vi "FaulhaberV3-Ascii_V1.vi"() -> (1 "searchnames":string[](array[string]), 2 "ID":u32[](array[numeric]), 3 "Faulhaber Objects":T3(array[cluster]))   [LabVIEW 2011] (continued)
of entries", "type"=enum."U8", "rw"=enum."ro", "lowLimit"="", "highLimit"="", "Default"="5", "Kommentart"=""}, {"ID"=594608129, "Name"="Trace buffer_Trace state", "type"=enum."U16", "rw"=enum."ro", "lowLimit"="", "highLimit"="", "Default"="", "Kommentart"=""}, {"ID"=594673664, "Name"="Logic trigger configuration_Number of entries", "type"=enum."U8", "rw"=enum."ro", "lowLimit"="", "highLimit"="", "Default"="2", "Kommentart"=""}, {"ID"=594673665, "Name"="Logic trigger configuration_Logic trigger AND mask", "type"=enum."U32", "rw"=enum."rw", "lowLimit"="0", "highLimit"="4294967295", "Default"="0x00", "Kommentart"=""}, {"ID"=594673666, "Name"="Logic trigger configuration_Logic trigger OR mask", "type"=enum."U32", "rw"=enum."rw", "lowLimit"="0", "highLimit"="4294967295", "Default"="0x00", "Kommentart"=""}, {"ID"=594739200, "Name"="Event trigger configuration_Number of entries", "type"=enum."U8", "rw"=enum."ro", "lowLimit"="", "highLimit"="", "Default"="1", "Kommentart"=""}, {"ID"=594739201, "Name"="Event trigger configuration_Event trigger event selection", "type"=enum."U16", "rw"=enum."unknown", "lowLimit"="", "highLimit"="", "Default"="", "Kommentart"=""}, {"ID"=594804736, "Name"="Event flag configuration_Number of entries", "type"=enum."U8", "rw"=enum."ro", "lowLimit"="", "highLimit"="", "Default"="2", "Kommentart"=""}, {"ID"=594804737, "Name"="Event flag configuration_Event flag set mask", "type"=enum."U16", "rw"=enum."rw", "lowLimit"="0", "highLimit"="65535", "Default"="0x0", "Kommentart"=""}, {"ID"=594804738, "Name"="Event flag configuration_Event flag reset mask", "type"=enum."U16", "rw"=enum."rw", "lowLimit"="0", "highLimit"="65535", "Default"="0x0", "Kommentart"=""}, {"ID"=595066880, "Name"="Trace channel configuration_Number of entries", "type"=enum."U8", "rw"=enum."ro", "lowLimit"="", "highLimit"="", "Default"="23", "Kommentart"=""}, {"ID"=595066881, "Name"="Trace channel configuration_Channel 1 filter time", "type"=enum."U16", "rw"=enum."rw", "lowLimit"="0", "highLimit"="65535", "Default"="0", "Kommentart"=""}, {"ID"=595066882, "Name"="Trace channel configuration_Channel 1 sample time", "type"=enum."U16", "rw"=enum."rw", "lowLimit"="0", "highLimit"="65535", "Default"="1", "Kommentart"=""}, {"ID"=595066883, "Name"="Trace channel configuration_Channel 1 number of samples", "type"=enum."U16", "rw"=enum."rw", "lowLimit"="0", "highLimit"="65535", "Default"="512", "Kommentart"=""}, {"ID"=595066884, "Name"="Trace channel configuration_Channel 1 monitoring values", "type"=enum."U16", "rw"=enum."rw", "lowLimit"="0", "highLimit"="0x003F", "Default"="0", "Kommentart"=""}, {"ID"=595066885, "Name"="Trace channel configuration_Channel 1 start event selection", "type"=enum."U8", "rw"=enum."unknown", "lowLimit"="", "highLimit"="", "Default"="", "Kommentart"=""}, {"ID"=595066886, "Name"="Trace channel configuration_Channel 1 update event selection", "type"=enum."U8", "rw"=enum."unknown", "lowLimit"="", "highLimit"="", "Default"="", "Kommentart"=""}, {"ID"=595066887, "Name"="Trace channel configuration_Channel 1 number of eval-cycles", "type"=enum."U32", "rw"=enum."rw", "lowLimit"="0", "highLimit"="4294967295", "Default"="0", "Kommentart"=""}, {"ID"=595066894, "Name"="Trace channel configuration_Channel 1 number of turnovers", "type"=enum."U32", "rw"=enum."ro", "lowLimit"="", "highLimit"="", "Default"="", "Kommentart"=""}, {"ID"=595066895, "Name"="Trace channel configuration_Channel 1 done", "type"=enum."U8", "rw"=enum."ro", "lowLimit"="", "highLimit"="", "Default"="", "Kommentart"=""}, {"ID"=595066896, "Name"="Trace channel configuration_Channel 1 abs min value", "type"=enum."S32", "rw"=enum."ro", "lowLimit"="", "highLimit"="", "Default"="2147483647", "Kommentart"=""}, {"ID"=595066897, "Name"="Trace channel configuration_Channel 1 abs max value", "type"=enum."S32", "rw"=enum."ro", "lowLimit"="", "highLimit"="", "Default"="-2147483648", "Kommentart"=""}, {"ID"=595066898, "Name"="Trace channel configuration_Channel 1 minimum", "type"=enum."S32", "rw"=enum."ro", "lowLimit"="", "highLimit"="", "Default"="", "Kommentart"=""}, {"ID"=595066899, "Name"="Trace channel configuration_Channel 1 maximum", "type"=enum."S32", "rw"=enum."ro", "lowLimit"="", "highLimit"="", "Default"="", "Kommentart"=""}, {"ID"=595066900, "Name"="Trace channel configuration_Channel 1 mean value", "type"=enum."S32", "rw"=enum."ro", "lowLimit"="", "highLimit"="", "Default"="", "Kommentart"=""}, {"ID"=595066901, "Name"="Trace channel configuration_Channel 1 rms value", "type"=enum."S32", "rw"=enum."ro", "lowLimit"="", "highLimit"="", "Default"="", "Kommentart"=""}, {"ID"=595066902, "Name"="Trace channel configuration_Channel 1 period time", "type"=enum."U32", "rw"=enum."ro", "lowLimit"="", "highLimit"="", "Default"="", "Kommentart"=""}, {"ID"=595066903, "Name"="Trace channel configuration_Channel 1 sigma", "type"=enum."S32", "rw"=enum."ro", "lowLimit"="", "highLimit"="", "Default"="", "Kommentart"=""}, {"ID"=595132416, "Name"="Trace channel configuration_Number of entries", "type"=enum."U8", "rw"=enum."ro", "lowLimit"="", "highLimit"="", "Default"="23", "Kommentart"=""}, {"ID"=595132417, "Name"="Trace channel configuration_Channel 2 filter time", "type"=enum."U16", "rw"=enum."rw", "lowLimit"="0", "highLimit"="65535", "Default"="0", "Kommentart"=""}, {"ID"=595132418, "Name"="Trace channel configuration_Channel 2 sample time", "type"=enum."U16", "rw"=enum."rw", "lowLimit"="0", "highLimit"="65535", "Default"="1", "Kommentart"=""}, {"ID"=595132419, "Name"="Trace channel configuration_Channel 2 number of samples", "type"=enum."U16", "rw"=enum."rw", "lowLimit"="0", "highLimit"="65535", "Default"="512", "Kommentart"=""}, {"ID"=595132420, "Name"="Trace channel configuration_Channel 2 monitoring values", "type"=enum."U16", "rw"=enum."rw", "lowLimit"="0", "highLimit"="0x003F", "Default"="0", "Kommentart"=""}, {"ID"=595132421, "Name"="Trace channel configuration_Channel 2 startevent selection", "type"=enum."U8", "rw"=enum."unknown", "lowLimit"="", "highLimit"="", "Default"="", "Kommentart"=""}, {"ID"=595132422, "Name"="Trace channel configuration_Channel 2 update event selection", "type"=enum."U8", "rw"=enum."unknown", "lowLimit"="", "highLimit"="", "Default"="", "Kommentart"=""}, {"ID"=595132423, "Name"="Trace channel configuration_Channel 2 number of eval-cycles", "type"=enum."U32", "rw"=enum."rw", "lowLimit"="0", "highLimit"="4294967295", "Default"="0", "Kommentart"=""}, {"ID"=595132430, "Name"="Trace channel configuration_Channel 2 number of turn-overs", "type"=enum."U32", "rw"=enum."ro", "lowLimit"="", "highLimit"="", "Default"="", "Kommentart"=""}, {"ID"=595132431, "Name"="Trace channel configuration_Channel 2 done", "type"=enum."U8", "rw"=enum."ro", "lowLimit"="", "highLimit"="", "Default"="", "Kommentart"=""}, {"ID"=595132432, "Name"="Trace channel configuration_Channel 2 abs min value", "type"=enum."S32", "rw"=enum."ro", "lowLimit"="", "highLimit"="", "Default"="2147483647", "Kommentart"=""}, {"ID"=595132433, "Name"="Trace channel configuration_Channel 2 abs max value", "type"=enum."S32", "rw"=enum."ro", "lowLimit"="", "highLimit"="", "Default"="-2147483648", "Kommentart"=""}, {"ID"=595132434, "Name"="Trace channel configuration_Channel 2 minimum", "type"=enum."S32", "rw"=enum."ro", "lowLimit"="", "highLimit"="", "Default"="", "Kommentart"=""}, {"ID"=595132435, "Name"="Trace channel configuration_Channel 2 maximum", "type"=enum."S32", "rw"=enum."ro", "lowLimit"="", "highLimit"="", "Default"="", "Kommentart"=""}, {"ID"=595132436, "Name"="Trace channel configuration_Channel 2 mean value", "type"=enum."S32", "rw"=enum."ro", "lowLimit"="", "highLimit"="", "Default"="", "Kommentart"=""}, {"ID"=595132437, "Name"="Trace channel configuration_Channel 2 rms value", "type"=enum."S32", "rw"=enum."ro", "lowLimit"="", "highLimit"="", "Default"="", "Kommentart"=""}, {"ID"=595132438, "Name"="Trace channel configuration_Channel 2 period time", "type"=enum."U32", "rw"=enum."ro", "lowLimit"="", "highLimit"="", "Default"="", "Kommentart"=""}, {"ID"=595132439, "Name"="Trace channel configuration_Channel 2 sigma", "type"=enum."S32", "rw"=enum."ro", "lowLimit"="", "highLimit"="", "Default"="", "Kommentart"=""}, {"ID"=595197952, "Name"="Trace channel configuration_Number of entries", "type"=enum."U8", "rw"=enum."ro", "lowLimit"="", "highLimit"="", "Default"="23", "Kommentart"=""}, {"ID"=595197953, "Name"="Trace channel configuration_Channel 3 filter time", "type"=enum."U16", "rw"=enum."rw", "lowLimit"="0", "highLimit"="65535", "Default"="0", "Kommentart"=""}, {"ID"=595197954, "Name"="Trace channel configuration_Channel 3 sample time", "type"=enum."U16", "rw"=enum."rw", "lowLimit"="0", "highLimit"="65535", "Default"="1", "Kommentart"=""}, {"ID"=595197955, "Name"="Trace channel configuration_Channel 3 number of samples", "type"=enum."U16", "rw"=enum."rw", "lowLimit"="0", "highLimit"="65535", "Default"="512", "Kommentart"=""}, {"ID"=595197956, "Name"="Trace channel configuration_Channel 3 monitoring values", "type"=enum."U16", "rw"=enum."rw", "lowLimit"="0", "highLimit"="0x003F", "Default"="0", "Kommentart"=""}, {"ID"=595197957, "Name"="Trace channel configuration_Channel 3 start event selection", "type"=enum."U8", "rw"=enum."unknown", "lowLimit"="", "highLimit"="", "Default"="", "Kommentart"=""}, {"ID"=595197958, "Name"="Trace channel configuration_Channel 3 update event selection", "type"=enum."U8", "rw"=enum."unknown", "lowLimit"="", "highLimit"="", "Default"="", "Kommentart"=""}, {"ID"=595197959, "Name"="Trace channel configuration_Channel 3 number of eval-cycles", "type"=enum."U32", "rw"=enum."rw", "lowLimit"="0", "highLimit"="4294967295", "Default"="0", "Kommentart"=""}, {"ID"=595197966, "Name"="Trace channel configuration_Channel 3 number of turn-overs", "type"=enum."U32", "rw"=enum."ro", "lowLimit"="", "highLimit"="", "Default"="", "Kommentart"=""}, {"ID"=595197967, "Name"="Trace channel configuration_Channel 3 done", "type"=enum."U8", "rw"=enum."ro", "lowLimit"="", "highLimit"="", "Default"="", "Kommentart"=""}, {"ID"=595197968, "Name"="Trace channel configuration_Channel 3 abs min value", "type"=enum."S32", "rw"=enum."ro", "lowLimit"="", "highLimit"="", "Default"="2147483647", "Kommentart"=""}, {"ID"=595197969, "Name"="Trace channel configuration_Channel 3 abs max value", "type"=enum."S32", "rw"=enum."ro", "lowLimit"="", "highLimit"="", "Default"="-2147483648", "Kommentart"=""}, {"ID"=595197970, "Name"="Trace channel configuration_Channel 3 minimum", "type"=enum."S32", "rw"=enum."ro", "lowLimit"="", "highLimit"="", "Default"="", "Kommentart"=""}, {"ID"=595197971, "Name"="Trace channel configuration_Channel 3 maximum", "type"=enum."S32", "rw"=enum."ro", "lowLimit"="", "highLimit"="", "Default"="", "Kommentart"=""}, {"ID"=595197972, "Name"="Trace channel configuration_Channel 3 mean value", "type"=enum."S32", "rw"=enum."ro", "lowLimit"="", "highLimit"="", "Default"="", "Kommentart"=""}, {"ID"=595197973, "Name"="Trace channel configuration_Channel 3 rms value", "type"=enum."S32", "rw"=enum."ro", "lowLimit"="", "highLimit"="", "Default"="", "Kommentart"=""}, {"ID"=595197974, "Name"="Trace channel configuration_Channel 3 period time", "type"=enum."U32", "rw"=enum."ro", "lowLimit"="", "highLimit"="", "Default"="", "Kommentart"=""}, {"ID"=595197975, "Name"="Trace channel configuration_Channel 3 sigma", "type"=enum."S32", "rw"=enum."ro", "lowLimit"="", "highLimit"="", "Default"="", "Kommentart"=""}, {"ID"=595263488, "Name"="Trace channel configuration_Number of entries", "type"=enum."U8", "rw"=enum."ro", "lowLimit"="", "highLimit"="", "Default"="23", "Kommentart"=""}, {"ID"=595263489, "Name"="Trace channel configuration_Channel 4 filter time", "type"=enum."U16", "rw"=enum."rw", "lowLimit"="0", "highLimit"="65535", "Default"="0", "Kommentart"=""}, {"ID"=595263490, "Name"="Trace channel configuration_Channel 4 sample time", "type"=enum."U16", "rw"=enum."rw", "lowLimit"="0", "highLimit"="65535", "Default"="1", "Kommentart"=""}, {"ID"=595263491, "Name"="Trace channel configuration_Channel 4 number of samples", "type"=enum."U16", "rw"=enum."rw", "lowLimit"="0", "highLimit"="65535", "Default"="512", "Kommentart"=""}, {"ID"=595263492, "Name"="Trace channel configuration_Channel 4 monitoring values", "type"=enum."U16", "rw"=enum."rw", "lowLimit"="0", "highLimit"="0x003F", "Default"="0", "Kommentart"=""}, {"ID"=595263493, "Name"="Trace channel configuration_Channel 4 start event selection", "type"=enum."U8", "rw"=enum."unknown", "lowLimit"="", "highLimit"="", "Default"="", "Kommentart"=""}, {"ID"=595263494, "Name"="Trace channel configuration_Channel 4 update event selection", "type"=enum."U8", "rw"=enum."unknown", "lowLimit"="", "highLimit"="", "Default"="", "Kommentart"=""}, {"ID"=595263495, "Name"="Trace channel configuration_Channel 4 number of eval-cycles", "type"=enum."U32", "rw"=enum."rw", "lowLimit"="0", "highLimit"="4294967295", "Default"="0", "Kommentart"=""}, {"ID"=595263502, "Name"="Trace channel configuration_Channel 4 number of turn-overs", "type"=enum."U32", "rw"=enum."ro", "lowLimit"="", "highLimit"="", "Default"="", "Kommentart"=""}, {"ID"=595263503, "Name"="Trace channel configuration_Channel 4 done", "type"=enum."U8", "rw"=enum."ro", "lowLimit"="", "highLimit"="", "Default"="", "Kommentart"=""}, {"ID"=595263504, "Name"="Trace channel configuration_Channel 4 abs min value", "type"=enum."S32", "rw"=enum."ro", "lowLimit"="", "highLimit"="", "Default"="2147483647", "Kommentart"=""}, {"ID"=595263505, "Name"="Trace channel configuration_Channel 4 abs max value", "type"=enum."S32", "rw"=enum."ro", "lowLimit"="", "highLimit"="", "Default"="-2147483648", "Kommentart"=""}, {"ID"=595263506, "Name"="Trace channel configuration_Channel 4 minimum", "type"=enum."S32", "rw"=enum."ro", "lowLimit"="", "highLimit"="", "Default"="", "Kommentart"=""}, {"ID"=595263507, "Name"="Trace channel configuration_Channel 4 maximum", "type"=enum."S32", "rw"=enum."ro", "lowLimit"="", "highLimit"="", "Default"="", "Kommentart"=""}, {"ID"=595263508, "Name"="Trace channel configuration_Channel 4 mean value", "type"=enum."S32", "rw"=enum."ro", "lowLimit"="", "highLimit"="", "Default"="", "Kommentart"=""}, {"ID"=595263509, "Name"="Trace channel configuration_Channel 4 rms value", "type"=enum."S32", "rw"=enum."ro", "lowLimit"="", "highLimit"="", "Default"="", "Kommentart"=""}, {"ID"=595263510, "Name"="Trace channel configuration_Channel 4 period time", "type"=enum."U32", "rw"=enum."ro", "lowLimit"="", "highLimit"="", "Default"="", "Kommentart"=""}, {"ID"=595263511, "Name"="Trace channel configuration_Channel 4 sigma", "type"=enum."S32", "rw"=enum."ro", "lowLimit"="", "highLimit"="", "Default"="", "Kommentart"=""}, {"ID"=595591168, "Name"="PRBS generator_Number of entries", "type"=enum."U8", "rw"=enum."ro", "lowLimit"="", "highLimit"="", "Default"="5", "Kommentart"=""}, {"ID"=595591169, "Name"="PRBS generator_Shift register init", "type"=enum."U16", "rw"=enum."rw", "lowLimit"="0", "highLimit"="65535", "Default"="", "Kommentart"=""}, {"ID"=595591170, "Name"="PRBS generator_Gain", "type"=enum."S16", "rw"=enum."rw", "lowLimit"="-32768", "highLimit"="32767", "Default"="", "Kommentart"=""}, {"ID"=595591171, "Name"="PRBS generator_Offset", "type"=enum."S16", "rw"=enum."rw", "lowLimit"="-32768", "highLimit"="32767", "Default"="", "Kommentart"=""}, {"ID"=595591172, "Name"="PRBS generator_Sample rate factor", "type"=enum."U8", "rw"=enum."rw", "lowLimit"="0", "highLimit"="255", "Default"="", "Kommentart"=""}, {"ID"=595591173, "Name"="PRBS generator_Enable", "type"=enum."U8", "rw"=enum."rw", "lowLimit"="0", "highLimit"="255", "Default"="", "Kommentart"=""}, {"ID"=595656704, "Name"="Start up generator_Number of entries", "type"=enum."U8", "rw"=enum."ro", "lowLimit"="", "highLimit"="", "Default"="8", "Kommentart"=""}, {"ID"=595656705, "Name"="Start up generator_Speed threshold", "type"=enum."U16", "rw"=enum."rw", "lowLimit"="0", "highLimit"="65535", "Default"="", "Kommentart"=""}, {"ID"=595656706, "Name"="Start up generator_Timeout time", "type"=enum."U32", "rw"=enum."rw", "lowLimit"="0", "highLimit"="4294967295", "Default"="", "Kommentart"=""}, {"ID"=595656707, "Name"="Start up generator_Target value", "type"=enum."U16", "rw"=enum."rw", "lowLimit"="0", "highLimit"="65535", "Default"="", "Kommentart"=""}, {"ID"=595656708, "Name"="Start up generator_Reset", "type"=enum."U8", "rw"=enum."rw", "lowLimit"="0", "highLimit"="255", "Default"="", "Kommentart"=""}, {"ID"=595656709, "Name"="Start up generator_Enable", "type"=enum."U8", "rw"=enum."rw", "lowLimit"="0", "highLimit"="255", "Default"="", "Kommentart"=""}, {"ID"=595656710, "Name"="Start up generator_Ready", "type"=enum."U32", "rw"=enum."rw", "lowLimit"="0", "highLimit"="4294967295", "Default"="", "Kommentart"=""}, {"ID"=595656711, "Name"="Start up generator_TimeThreshold", "type"=enum."U32", "rw"=enum."rw", "lowLimit"="0", "highLimit"="4294967295", "Default"="", "Kommentart"=""}, {"ID"=595656712, "Name"="Start up generator_Iteration", "type"=enum."U32", "rw"=enum."rw", "lowLimit"="0", "highLimit"="4294967295", "Default"="", "Kommentart"=""}, {"ID"=595722240, "Name"="Sinusoidal excitation_Number of entries", "type"=enum."U8", "rw"=enum."ro", "lowLimit"="", "highLimit"="", "Default"="3", "Kommentart"=""}, {"ID"=595722241, "Name"="Sinusoidal excitation_Amplitude", "type"=enum."U16", "rw"=enum."rw", "lowLimit"="0", "highLimit"="65535", "Default"="", "Kommentart"=""}, {"ID"=595722242, "Name"="Sinusoidal excitation_Frequency", "type"=enum."U16", "rw"=enum."rw", "lowLimit"="0", "highLimit"="65535", "Default"="", "Kommentart"=""}, {"ID"=595722243, "Name"="Sinusoidal excitation_Enable", "type"=enum."U8", "rw"=enum."rw", "lowLimit"="0", "highLimit"="255", "Default"="", "Kommentart"=""}, {"ID"=596574208, "Name"="Select signal generator source_Number of entries", "type"=enum."U8", "rw"=enum."ro", "lowLimit"="", "highLimit"="", "Default"="1", "Kommentart"=""}, {"ID"=596574209, "Name"="Select signal generator source_Selector", "type"=enum."U8", "rw"=enum."rw", "lowLimit"="0", "highLimit"="255", "Default"="0", "Kommentart"=""}, {"ID"=602931200, "Name"="23F0_00_Number of entries", "type"=enum."U8", "rw"=enum."ro", "lowLimit"="", "highLimit"="", "Default"="6", "Kommentart"=""}, {"ID"=602931201, "Name"="23F0_00_23F0_01", "type"=enum."U32", "rw"=enum."ro", "lowLimit"="", "highLimit"="", "Default"="", "Kommentart"=""}, {"ID"=602931202, "Name"="23F0_00_23F0_02", "type"=enum."U8", "rw"=enum."ro", "lowLimit"="", "highLimit"="", "Default"="", "Kommentart"=""}, {"ID"=602931203, "Name"="23F0_00_23F0_03", "type"=enum."U8", "rw"=enum."ro", "lowLimit"="", "highLimit"="", "Default"="", "Kommentart"=""}, {"ID"=602931204, "Name"="23F0_00_23F0_04", "type"=enum."U16", "rw"=enum."ro", "lowLimit"="", "highLimit"="", "Default"="", "Kommentart"=""}, {"ID"=602931205, "Name"="23F0_00_23F0_05", "type"=enum."U32", "rw"=enum."ro", "lowLimit"="", "highLimit"="", "Default"="", "Kommentart"=""}, {"ID"=602931206, "Name"="23F0_00_23F0_06", "type"=enum."U32", "rw"=enum."ro", "lowLimit"="", "highLimit"="", "Default"="", "Kommentart"=""}, {"ID"=602996736, "Name"="23F1_00_Number of entries", "type"=enum."U8", "rw"=enum."ro", "lowLimit"="", "highLimit"="", "Default"="2", "Kommentart"=""}, {"ID"=602996737, "Name"="23F1_00_23F1_01", "type"=enum."S32", "rw"=enum."ro", "lowLimit"="", "highLimit"="", "Default"="", "Kommentart"=""}, {"ID"=602996738, "Name"="23F1_00_23F1_02", "type"=enum."S32", "rw"=enum."ro", "lowLimit"="", "highLimit"="", "Default"="", "Kommentart"=""}, {"ID"=603127808, "Name"="23F2_00 _Number of entries", "type"=enum."U8", "rw"=enum."ro", "lowLimit"="", "highLimit"="", "Default"="5", "Kommentart"=""}, {"ID"=603127809, "Name"="23F2_00 _Actual state", "type"=enum."S8", "rw"=enum."ro", "lowLimit"="", "highLimit"="", "Default"="", "Kommentart"=""}, {"ID"=603127810, "Name"="23F2_00 _Demand position", "type"=enum."S32", "rw"=enum."ro", "lowLimit"="", "highLimit"="", "Default"="", "Kommentart"=""}, {"ID"=603127811, "Name"="23F2_00 _Demand speed", "type"=enum."S32", "rw"=enum."ro", "lowLimit"="", "highLimit"="", "Default"="", "Kommentart"=""}, {"ID"=603127812, "Name"="23F2_00 _Demand acceleration", "type"=enum."S16", "rw"=enum."ro", "lowLimit"="", "highLimit"="", "Default"="", "Kommentart"=""}, {"ID"=603127813, "Name"="23F2_00 _Initial state", "type"=enum."S8", "rw"=enum."ro", "lowLimit"="", "highLimit"="", "Default"="", "Kommentart"=""}, {"ID"=603979776, "Name"="Communication parameters_Number of entries", "type"=enum."U8", "rw"=enum."ro", "lowLimit"="", "highLimit"="", "Default"="7", "Kommentart"=""}, {"ID"=603979777, "Name"="Communication parameters_CAN rate", "type"=enum."U8", "rw"=enum."unknown", "lowLimit"="", "highLimit"="", "Default"="", "Kommentart"=""}, {"ID"=603979778, "Name"="Communication parameters_RS232 rate", "type"=enum."U8", "rw"=enum."unknown", "lowLimit"="", "highLimit"="", "Default"="", "Kommentart"=""}, {"ID"=603979779, "Name"="Communication parameters_Node ID", "type"=enum."U8", "rw"=enum."rw", "lowLimit"="1", "highLimit"="127", "Default"="1", "Kommentart"=""}, {"ID"=603979780, "Name"="Communication parameters_Communication settings", "type"=enum."U32", "rw"=enum."rw", "lowLimit"="0", "highLimit"="0x00078303", "Default"="0x00030302", "Kommentart"=""}, {"ID"=603979781, "Name"="Communication parameters_RS232 NetMode", "type"=enum."U8", "rw"=enum."rw", "lowLimit"="0", "highLimit"="255", "Default"="0", "Kommentart"=""}, {"ID"=603979782, "Name"="Communication parameters_ComState", "type"=enum."U16", "rw"=enum."ro", "lowLimit"="", "highLimit"="", "Default"="", "Kommentart"=""}, {"ID"=603979783, "Name"="Communication parameters_ErrState", "type"=enum."U16", "rw"=enum."ro", "lowLimit"="", "highLimit"="", "Default"="", "Kommentart"=""}, {"ID"=604045312, "Name"="USB Delay", "type"=enum."U8", "rw"=enum."wo", "lowLimit"="0", "highLimit"="255", "Default"="5", "Kommentart"=""}, {"ID"=604241920, "Name"="FAID", "type"=enum."U16", "rw"=enum."wo", "lowLimit"="0", "highLimit"="65535", "Default"="0", "Kommentart"=""}, {"ID"=604307456, "Name"="Bootloader SW version", "type"=enum."string", "rw"=enum."ro", "lowLimit"="", "highLimit"="", "Default"="0", "Kommentart"=""}, {"ID"=604372992, "Name"="OD revision number", "type"=enum."U32", "rw"=enum."ro", "lowLimit"="", "highLimit"="", "Default"="", "Kommentart"=""}, {"ID"=604438528, "Name"="SW revision number", "type"=enum."U32", "rw"=enum."ro", "lowLimit"="", "highLimit"="", "Default"="", "Kommentart"=""}, {"ID"=604504064, "Name"="XDC Number", "type"=enum."U32", "rw"=enum."ro", "lowLimit"="", "highLimit"="", "Default"="", "Kommentart"=""}, {"ID"=605028352, "Name"="CAL access_Number of entries", "type"=enum."U8", "rw"=enum."ro", "lowLimit"="", "highLimit"="", "Default"="1", "Kommentart"=""}, {"ID"=605028353, "Name"="CAL access_CAL key", "type"=enum."U32", "rw"=enum."rw", "lowLimit"="0", "highLimit"="4294967295", "Default"="", "Kommentart"=""}, {"ID"=620756992, "Name"="ADC scaling (offset|gain)_Number of entries", "type"=enum."U8", "rw"=enum."ro", "lowLimit"="", "highLimit"="", "Default"="14", "Kommentart"=""}, {"ID"=620756993, "Name"="ADC scaling (offset|gain)_IA scaling", "type"=enum."U32", "rw"=enum."ro", "lowLimit"="0x0", "highLimit"="", "Default"="", "Kommentart"=""}, {"ID"=620756994, "Name"="ADC scaling (offset|gain)_IB scaling", "type"=enum."U32", "rw"=enum."ro", "lowLimit"="0x0", "highLimit"="", "Default"="", "Kommentart"=""}, {"ID"=620756995, "Name"="ADC scaling (offset|gain)_IC scaling", "type"=enum."U32", "rw"=enum."ro", "lowLimit"="0x0", "highLimit"="", "Default"="", "Kommentart"=""}, {"ID"=620756996, "Name"="ADC scaling (offset|gain)_Hall A scaling", "type"=enum."U32", "rw"=enum."ro", "lowLimit"="0x0", "highLimit"="", "Default"="", "Kommentart"=""}, {"ID"=620756997, "Name"="ADC scaling (offset|gain)_Hall B scaling", "type"=enum."U32", "rw"=enum."ro", "lowLimit"="0x0", "highLimit"="", "Default"="", "Kommentart"=""}, {"ID"=620756998, "Name"="ADC scaling (offset|gain)_Hall C scaling", "type"=enum."U32", "rw"=enum."ro", "lowLimit"="0x0", "highLimit"="", "Default"="", "Kommentart"=""}, {"ID"=620756999, "Name"="ADC scaling (offset|gain)_Analog input 1 scaling", "type"=enum."U32", "rw"=enum."ro", "lowLimit"="0x0", "highLimit"="", "Default"="", "Kommentart"=""}, {"ID"=620757000, "Name"="ADC scaling (offset|gain)_Analog input 2 scaling", "type"=enum."U32", "rw"=enum."ro", "lowLimit"="0x0", "highLimit"="", "Default"="", "Kommentart"=""}, {"ID"=620757001, "Name"="ADC scaling (offset|gain)_Uel scaling", "type"=enum."U32", "rw"=enum."ro", "lowLimit"="0x0", "highLimit"="", "Default"="", "Kommentart"=""}, {"ID"=620757002, "Name"="ADC scaling (offset|gain)_Udc scaling", "type"=enum."U32", "rw"=enum."ro", "lowLimit"="0x0", "highLimit"="", "Default"="", "Kommentart"=""}, {"ID"=620757003, "Name"="ADC scaling (offset|gain)_Internal temperature scaling", "type"=enum."U32", "rw"=enum."ro", "lowLimit"="0x0", "highLimit"="", "Default"="", "Kommentart"=""}, {"ID"=620757004, "Name"="ADC scaling (offset|gain)_External temperature scaling", "type"=enum."U32", "rw"=enum."ro", "lowLimit"="0x0", "highLimit"="", "Default"="", "Kommentart"=""}, {"ID"=620757005, "Name"="ADC scaling (offset|gain)_Motor NTC gain", "type"=enum."S32", "rw"=enum."ro", "lowLimit"="0x80000000", "highLimit"="", "Default"="", "Kommentart"=""}, {"ID"=620757006, "Name"="ADC scaling (offset|gain)_Motor NTC offset", "type"=enum."S16", "rw"=enum."ro", "lowLimit"="0xFFFF8000", "highLimit"="", "Default"="", "Kommentart"=""}, {"ID"=620822528, "Name"="Hall scaling_Number of entries", "type"=enum."U8", "rw"=enum."ro", "lowLimit"="", "highLimit"="", "Default"="14", "Kommentart"=""}, {"ID"=620822529, "Name"="Hall scaling_Gain A", "type"=enum."U16", "rw"=enum."ro", "lowLimit"="", "highLimit"="", "Default"="", "Kommentart"=""}, {"ID"=620822530, "Name"="Hall scaling_Hall A  offset", "type"=enum."U16", "rw"=enum."ro", "lowLimit"="", "highLimit"="", "Default"="", "Kommentart"=""}, {"ID"=620822531, "Name"="Hall scaling_Hall A sin", "type"=enum."U16", "rw"=enum."ro", "lowLimit"="", "highLimit"="", "Default"="", "Kommentart"=""}, {"ID"=620822532, "Name"="Hall scaling_Hall A cos", "type"=enum."U16", "rw"=enum."ro", "lowLimit"="", "highLimit"="", "Default"="", "Kommentart"=""}, {"ID"=620822533, "Name"="Hall scaling_Corr A", "type"=enum."U16", "rw"=enum."ro", "lowLimit"="", "highLimit"="", "Default"="", "Kommentart"=""}, {"ID"=620822534, "Name"="Hall scaling_Hall B offset", "type"=enum."U16", "rw"=enum."ro", "lowLimit"="", "highLimit"="", "Default"="", "Kommentart"=""}, {"ID"=620822535, "Name"="Hall scaling_Hall B sin", "type"=enum."U16", "rw"=enum."ro", "lowLimit"="", "highLimit"="", "Default"="", "Kommentart"=""}, {"ID"=620822536, "Name"="Hall scaling_Hall B cos", "type"=enum."U16", "rw"=enum."ro", "lowLimit"="", "highLimit"="", "Default"="", "Kommentart"=""}, {"ID"=620822537, "Name"="Hall scaling_Corr B", "type"=enum."U16", "rw"=enum."ro", "lowLimit"="", "highLimit"="", "Default"="", "Kommentart"=""}, {"ID"=620822538, "Name"="Hall scaling_Hall C offset", "type"=enum."U16", "rw"=enum."ro", "lowLimit"="", "highLimit"="", "Default"="", "Kommentart"=""}, {"ID"=620822539, "Name"="Hall scaling_Hall C sin", "type"=enum."U16", "rw"=enum."ro", "lowLimit"="", "highLimit"="", "Default"="", "Kommentart"=""}, {"ID"=620822540, "Name"="Hall scaling_Hall C cos", "type"=enum."U16", "rw"=enum."ro", "lowLimit"="", "highLimit"="", "Default"="", "Kommentart"=""}, {"ID"=620822541, "Name"="Hall scaling_Offset A", "type"=enum."U16", "rw"=enum."ro", "lowLimit"="", "highLimit"="", "Default"="", "Kommentart"=""}, {"ID"=620822542, "Name"="Hall scaling_Offset B", "type"=enum."U16", "rw"=enum."ro", "lowLimit"="", "highLimit"="", "Default"="", "Kommentart"=""}, {"ID"=620888064, "Name"="Internal filter parameters_Number of entries", "type"=enum."U8", "rw"=enum."ro", "lowLimit"="", "highLimit"="", "Default"="13", "Kommentart"=""}, {"ID"=620888065, "Name"="Internal filter parameters_Filter time actual velocity", "type"=enum."U16", "rw"=enum."rw", "lowLimit"="0", "highLimit"="65535", "Default"="256", "Kommentart"=""}, {"ID"=620888066, "Name"="Internal filter parameters_Filter time IA ", "type"=enum."U16", "rw"=enum."ro", "lowLimit"="", "highLimit"="", "Default"="", "Kommentart"=""}, {"ID"=620888067, "Name"="Internal filter parameters_Filter time IB", "type"=enum."U16", "rw"=enum."ro", "lowLimit"="", "highLimit"="", "Default"="", "Kommentart"=""}, {"ID"=620888068, "Name"="Internal filter parameters_Filter time IC", "type"=enum."U16", "rw"=enum."ro", "lowLimit"="", "highLimit"="", "Default"="", "Kommentart"=""}, {"ID"=620888069, "Name"="Internal filter parameters_Filter time Uel", "type"=enum."U16", "rw"=enum."ro", "lowLimit"="", "highLimit"="", "Default"="", "Kommentart"=""}, {"ID"=620888070, "Name"="Internal filter parameters_Filter time Umot", "type"=enum."U16", "rw"=enum."ro", "lowLimit"="", "highLimit"="", "Default"="", "Kommentart"=""}, {"ID"=620888071, "Name"="Internal filter parameters_Additional filter time Uel", "type"=enum."U16", "rw"=enum."ro", "lowLimit"="0x0", "highLimit"="", "Default"="", "Kommentart"=""}, {"ID"=620888072, "Name"="Internal filter parameters_Additional filter time Umot", "type"=enum."U16", "rw"=enum."ro", "lowLimit"="0x0", "highLimit"="", "Default"="", "Kommentart"=""}, {"ID"=620888073, "Name"="Internal filter parameters_Filter time Iq thermal model", "type"=enum."U16", "rw"=enum."ro", "lowLimit"="", "highLimit"="", "Default"="", "Kommentart"=""}, {"ID"=620888074, "Name"="Internal filter parameters_Filter time Id thermal model", "type"=enum."U16", "rw"=enum."ro", "lowLimit"="", "highLimit"="", "Default"="", "Kommentart"=""}, {"ID"=620888075, "Name"="Internal filter parameters_Filter time Imot thermal model", "type"=enum."U16", "rw"=enum."ro", "lowLimit"="", "highLimit"="", "Default"="", "Kommentart"=""}, {"ID"=620888076, "Name"="Internal filter parameters_Filter time setpoint voltage model", "type"=enum."U16", "rw"=enum."ro", "lowLimit"="", "highLimit"="", "Default"="", "Kommentart"=""}, {"ID"=620888077, "Name"="Internal filter parameters_Filter time electrical time constant", "type"=enum."U16", "rw"=enum."rw", "lowLimit"="0", "highLimit"="65535", "Default"="", "Kommentart"=""}, {"ID"=620953600, "Name"="Boot options", "type"=enum."U16", "rw"=enum."rw", "lowLimit"="0", "highLimit"="2", "Default"="1", "Kommentart"=""}, {"ID"=621019136, "Name"="Hall compensation_Number of entries", "type"=enum."U8", "rw"=enum."ro", "lowLimit"="", "highLimit"="", "Default"="12", "Kommentart"=""}, {"ID"=621019137, "Name"="Hall compensation_Entry 01", "type"=enum."S16", "rw"=enum."ro", "lowLimit"="", "highLimit"="", "Default"="", "Kommentart"=""}, {"ID"=621019138, "Name"="Hall compensation_Entry 02", "type"=enum."S16", "rw"=enum."ro", "lowLimit"="", "highLimit"="", "Default"="", "Kommentart"=""}, {"ID"=621019139, "Name"="Hall compensation_Entry 03", "type"=enum."S16", "rw"=enum."ro", "lowLimit"="", "highLimit"="", "Default"="", "Kommentart"=""}, {"ID"=621019140, "Name"="Hall compensation_Entry 04", "type"=enum."S16", "rw"=enum."ro", "lowLimit"="", "highLimit"="", "Default"="", "Kommentart"=""}, {"ID"=621019141, "Name"="Hall compensation_Entry 05", "type"=enum."S16", "rw"=enum."ro", "lowLimit"="", "highLimit"="", "Default"="", "Kommentart"=""}, {"ID"=621019142, "Name"="Hall compensation_Entry 06", "type"=enum."S16", "rw"=enum."ro", "lowLimit"="", "highLimit"="", "Default"="", "Kommentart"=""}, {"ID"=621019143, "Name"="Hall compensation_Entry 07", "type"=enum."S16", "rw"=enum."ro", "lowLimit"="", "highLimit"="", "Default"="", "Kommentart"=""}, {"ID"=621019144, "Name"="Hall compensation_Entry 08", "type"=enum."S16", "rw"=enum."ro", "lowLimit"="", "highLimit"="", "Default"="", "Kommentart"=""}, {"ID"=621019145, "Name"="Hall compensation_Entry 09", "type"=enum."S16", "rw"=enum."ro", "lowLimit"="", "highLimit"="", "Default"="", "Kommentart"=""}, {"ID"=621019146, "Name"="Hall compensation_Entry 10", "type"=enum."S16", "rw"=enum."ro", "lowLimit"="", "highLimit"="", "Default"="", "Kommentart"=""}, {"ID"=621019147, "Name"="Hall compensation_Entry 11", "type"=enum."S16", "rw"=enum."ro", "lowLimit"="", "highLimit"="", "Default"="", "Kommentart"=""}, {"ID"=621019148, "Name"="Hall compensation_Entry 12", "type"=enum."S16", "rw"=enum."ro", "lowLimit"="", "highLimit"="", "Default"="", "Kommentart"=""}, {"ID"=621150208, "Name"="Encoder compensation_Number of entries", "type"=enum."U8", "rw"=enum."ro", "lowLimit"="", "highLimit"="", "Default"="64", "Kommentart"=""}, {"ID"=621150209, "Name"="Encoder compensation_Value 0", "type"=enum."S16", "rw"=enum."rw", "lowLimit"="-32768", "highLimit"="32767", "Default"="0", "Kommentart"=""}, {"ID"=621150210, "Name"="Encoder compensation_Value 1", "type"=enum."S16", "rw"=enum."rw", "lowLimit"="-32768", "highLimit"="32767", "Default"="0", "Kommentart"=""}, {"ID"=621150211, "Name"="Encoder compensation_Value 2", "type"=enum."S16", "rw"=enum."rw", "lowLimit"="-32768", "highLimit"="32767", "Default"="0", "Kommentart"=""}, {"ID"=621150212, "Name"="Encoder compensation_Value 3", "type"=enum."S16", "rw"=enum."rw", "lowLimit"="-32768", "highLimit"="32767", "Default"="0", "Kommentart"=""}, {"ID"=621150213, "Name"="Encoder compensation_Value 4", "type"=enum."S16", "rw"=enum."rw", "lowLimit"="-32768", "highLimit"="32767", "Default"="0", "Kommentart"=""}, {"ID"=621150214, "Name"="Encoder compensation_Value 5", "type"=enum."S16", "rw"=enum."rw", "lowLimit"="-32768", "highLimit"="32767", "Default"="0", "Kommentart"=""}, {"ID"=621150215, "Name"="Encoder compensation_Value 6", "type"=enum."S16", "rw"=enum."rw", "lowLimit"="-32768", "highLimit"="32767", "Default"="0", "Kommentart"=""}, {"ID"=621150216, "Name"="Encoder compensation_Value 7", "type"=enum."S16", "rw"=enum."rw", "lowLimit"="-32768", "highLimit"="32767", "Default"="0", "Kommentart"=""}, {"ID"=621150217, "Name"="Encoder compensation_Value 8", "type"=enum."S16", "rw"=enum."rw", "lowLimit"="-32768", "highLimit"="32767", "Default"="0", "Kommentart"=""}, {"ID"=621150218, "Name"="Encoder compensation_Value 9", "type"=enum."S16", "rw"=enum."rw", "lowLimit"="-32768", "highLimit"="32767", "Default"="0", "Kommentart"=""}, {"ID"=621150219, "Name"="Encoder compensation_Value 10", "type"=enum."S16", "rw"=enum."rw", "lowLimit"="-32768", "highLimit"="32767", "Default"="0", "Kommentart"=""}, {"ID"=621150220, "Name"="Encoder compensation_Value 11", "type"=enum."S16", "rw"=enum."rw", "lowLimit"="-32768", "highLimit"="32767", "Default"="0", "Kommentart"=""}, {"ID"=621150221, "Name"="Encoder compensation_Value 12", "type"=enum."S16", "rw"=enum."rw", "lowLimit"="-32768", "highLimit"="32767", "Default"="0", "Kommentart"=""}, {"ID"=621150222, "Name"="Encoder compensation_Value 13", "type"=enum."S16", "rw"=enum."rw", "lowLimit"="-32768", "highLimit"="32767", "Default"="0", "Kommentart"=""}, {"ID"=621150223, "Name"="Encoder compensation_Value 14", "type"=enum."S16", "rw"=enum."rw", "lowLimit"="-32768", "highLimit"="32767", "Default"="0", "Kommentart"=""}, {"ID"=621150224, "Name"="Encoder compensation_Value 15", "type"=enum."S16", "rw"=enum."rw", "lowLimit"="-32768", "highLimit"="32767", "Default"="0", "Kommentart"=""}, {"ID"=621150225, "Name"="Encoder compensation_Value 16", "type"=enum."S16", "rw"=enum."rw", "lowLimit"="-32768", "highLimit"="32767", "Default"="0", "Kommentart"=""}, {"ID"=621150226, "Name"="Encoder compensation_Value 17", "type"=enum."S16", "rw"=enum."rw", "lowLimit"="-32768", "highLimit"="32767", "Default"="0", "Kommentart"=""}, {"ID"=621150227, "Name"="Encoder compensation_Value 18", "type"=enum."S16", "rw"=enum."rw", "lowLimit"="-32768", "highLimit"="32767", "Default"="0", "Kommentart"=""}, {"ID"=621150228, "Name"="Encoder compensation_Value 19", "type"=enum."S16", "rw"=enum."rw", "lowLimit"="-32768", "highLimit"="32767", "Default"="0", "Kommentart"=""}, {"ID"=621150229, "Name"="Encoder compensation_Value 20", "type"=enum."S16", "rw"=enum."rw", "lowLimit"="-32768", "highLimit"="32767", "Default"="0", "Kommentart"=""}, {"ID"=621150230, "Name"="Encoder compensation_Value 21", "type"=enum."S16", "rw"=enum."rw", "lowLimit"="-32768", "highLimit"="32767", "Default"="0", "Kommentart"=""}, {"ID"=621150231, "Name"="Encoder compensation_Value 22", "type"=enum."S16", "rw"=enum."rw", "lowLimit"="-32768", "highLimit"="32767", "Default"="0", "Kommentart"=""}, {"ID"=621150232, "Name"="Encoder compensation_Value 23", "type"=enum."S16", "rw"=enum."rw", "lowLimit"="-32768", "highLimit"="32767", "Default"="0", "Kommentart"=""}, {"ID"=621150233, "Name"="Encoder compensation_Value 24", "type"=enum."S16", "rw"=enum."rw", "lowLimit"="-32768", "highLimit"="32767", "Default"="0", "Kommentart"=""}, {"ID"=621150234, "Name"="Encoder compensation_Value 25", "type"=enum."S16", "rw"=enum."rw", "lowLimit"="-32768", "highLimit"="32767", "Default"="0", "Kommentart"=""}, {"ID"=621150235, "Name"="Encoder compensation_Value 26", "type"=enum."S16", "rw"=enum."rw", "lowLimit"="-32768", "highLimit"="32767", "Default"="0", "Kommentart"=""}, {"ID"=621150236, "Name"="Encoder compensation_Value 27", "type"=enum."S16", "rw"=enum."rw", "lowLimit"="-32768", "highLimit"="32767", "Default"="0", "Kommentart"=""}, {"ID"=621150237, "Name"="Encoder compensation_Value 28", "type"=enum."S16", "rw"=enum."rw", "lowLimit"="-32768", "highLimit"="32767", "Default"="0", "Kommentart"=""}, {"ID"=621150238, "Name"="Encoder compensation_Value 29", "type"=enum."S16", "rw"=enum."rw", "lowLimit"="-32768", "highLimit"="32767", "Default"="0", "Kommentart"=""}, {"ID"=621150239, "Name"="Encoder compensation_Value 30", "type"=enum."S16", "rw"=enum."rw", "lowLimit"="-32768", "highLimit"="32767", "Default"="0", "Kommentart"=""}, {"ID"=621150240, "Name"="Encoder compensation_Value 31", "type"=enum."S16", "rw"=enum."rw", "lowLimit"="-32768", "highLimit"="32767", "Default"="0", "Kommentart"=""}, {"ID"=621150241, "Name"="Encoder compensation_Value 32", "type"=enum."S16", "rw"=enum."rw", "lowLimit"="-32768", "highLimit"="32767", "Default"="0", "Kommentart"=""}, {"ID"=621150242, "Name"="Encoder compensation_Value 33", "type"=enum."S16", "rw"=enum."rw", "lowLimit"="-32768", "highLimit"="32767", "Default"="0", "Kommentart"=""}, {"ID"=621150243, "Name"="Encoder compensation_Value 34", "type"=enum."S16", "rw"=enum."rw", "lowLimit"="-32768", "highLimit"="32767", "Default"="0", "Kommentart"=""}, {"ID"=621150244, "Name"="Encoder compensation_Value 35", "type"=enum."S16", "rw"=enum."rw", "lowLimit"="-32768", "highLimit"="32767", "Default"="0", "Kommentart"=""}, {"ID"=621150245, "Name"="Encoder compensation_Value 36", "type"=enum."S16", "rw"=enum."rw", "lowLimit"="-32768", "highLimit"="32767", "Default"="0", "Kommentart"=""}, {"ID"=621150246, "Name"="Encoder compensation_Value 37", "type"=enum."S16", "rw"=enum."rw", "lowLimit"="-32768", "highLimit"="32767", "Default"="0", "Kommentart"=""}, {"ID"=621150247, "Name"="Encoder compensation_Value 38", "type"=enum."S16", "rw"=enum."rw", "lowLimit"="-32768", "highLimit"="32767", "Default"="0", "Kommentart"=""}, {"ID"=621150248, "Name"="Encoder compensation_Value 39", "type"=enum."S16", "rw"=enum."rw", "lowLimit"="-32768", "highLimit"="32767", "Default"="0", "Kommentart"=""}, {"ID"=621150249, "Name"="Encoder compensation_Value 40", "type"=enum."S16", "rw"=enum."rw", "lowLimit"="-32768", "highLimit"="32767", "Default"="0", "Kommentart"=""}, {"ID"=621150250, "Name"="Encoder compensation_Value 41", "type"=enum."S16", "rw"=enum."rw", "lowLimit"="-32768", "highLimit"="32767", "Default"="0", "Kommentart"=""}, {"ID"=621150251, "Name"="Encoder compensation_Value 42", "type"=enum."S16", "rw"=enum."rw", "lowLimit"="-32768", "highLimit"="32767", "Default"="0", "Kommentart"=""}, {"ID"=621150252, "Name"="Encoder compensation_Value 43", "type"=enum."S16", "rw"=enum."rw", "lowLimit"="-32768", "highLimit"="32767", "Default"="0", "Kommentart"=""}, {"ID"=621150253, "Name"="Encoder compensation_Value 44", "type"=enum."S16", "rw"=enum."rw", "lowLimit"="-32768", "highLimit"="32767", 
